vi "BoundsToRect32.vi"(1 "Offset (0,0)":T1, 2 "Bounds":T1) -> (0 "Rect32":T3)   [LabVIEW 2020, in "NI_XNodeSupport.lvlib"]
uses:
  NI_XNodeSupport.lvlib
  XNodeRect32.ctl
  XNodeInt.ctl
  XNodeBounds.ctl
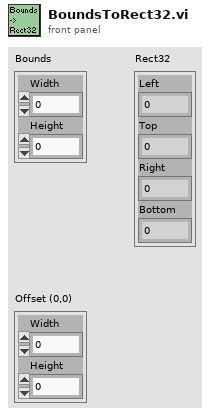
[diagram p1: front panel]
types:
  T1 = typedef "NI_XNodeSupport.lvlib/XNodeBounds.ctl" = cluster{"Width":T2, "Height":T2}
  T2 = typedef "NI_XNodeSupport.lvlib/XNodeInt.ctl" = i32
  T3 = typedef "NI_XNodeSupport.lvlib/XNodeRect32.ctl" = cluster{"Left":T2, "Top":T2, "Right":T2, "Bottom":T2}
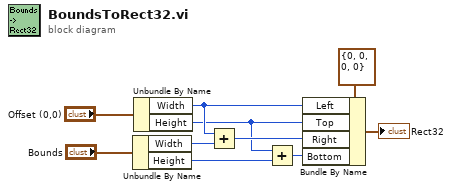
[diagram p0: block diagram]
diagram:
  n1 = Unbundle By Name("Bounds") -> ("Width"=w6:T2, "Height"=w3:T2)
  n2 = Unbundle By Name("Offset (0,0)") -> ("Width"=w7:T2, "Height"=w4:T2)
  n3 = Add(x=w7, y=w6) -> (x+y=w5:T2)
  n4 = Add(x=w4, y=w3) -> (x+y=w2:T2)
  n5 = Bundle By Name(cluster=T3 {"Left"=0, "Top"=0, "Right"=0, "Bottom"=0} ("Rect32"), "Left"=w7, "Top"=w4, "Right"=w5, "Bottom"=w2) -> (→"Rect32":T3)
